vi "float_binread.vi"(8 "エラー入力（エラーなし）":errorcluster, 10 "offset":i64, 11 "バイトストリームファイル入力":refnum<file>) -> (0 "エラー出力":errorcluster, 2 "float":sgl, 3 "バイトストリームファイル出力":refnum<file>)   [LabVIEW 2015]
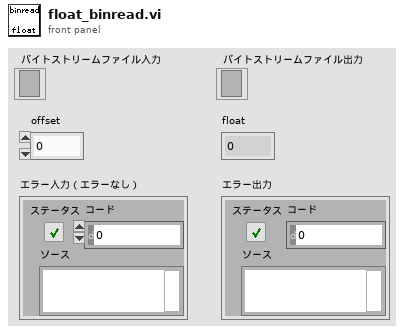
[diagram p1: front panel]
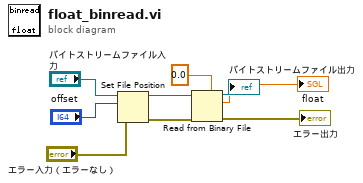
[diagram p0: block diagram]
diagram:
  n1 = Set File Position(offset (in bytes) (0)="offset", refnum="バイトストリームファイル入力", error in="エラー入力（エラーなし）") -> (refnum out=w2:refnum<file>, error out=w3:errorcluster)  [unwired: 1 in]
  n2 = Read from Binary File(5:sgl 0.0, 8:w3, 11:w2) -> (0:→"エラー出力":errorcluster, 2:→"float":sgl, 3:→"バイトストリームファイル出力":refnum<file>)  [unwired: 3 in, 1 out]
